vi "LuaVIEW Pull (refnum).vi"(5 "LuaVIEW reference in":T1, 11 "error in (no error)":errorcluster) -> (4 "refnum":refnum<vi>, 6 "LuaVIEW reference out":T1, 15 "error out":errorcluster)   [LabVIEW 2013]
doc: "Retrieves a refnum data item from the head/bottom of the Lua stack and removes it, thereby shifting any remaining data items down by one. The returned value is a generic refnum that identifies some LabVIEW side object and must be cast to the appropriate type before use. This VI is part of a polymorphic set that supports the pulling various data types. To change the type being pulled, pop up on this VI's diagram icon and use the \"Select Type\" sub menu."
uses:
  typedefs/t_LuaVIEW Reference.ctl
  typedefs/et_LuaVIEW CIN Actions.ctl
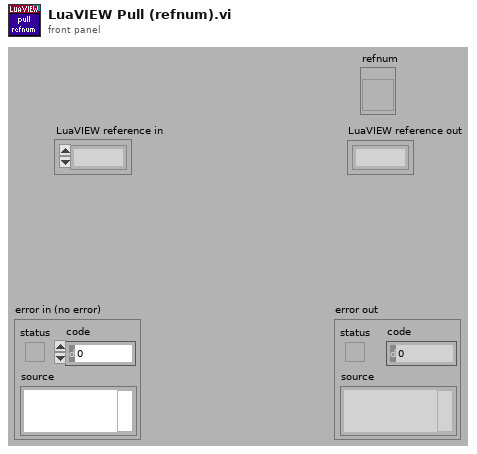
[diagram p1: front panel]
types:
  T1 = typedef "t_LuaVIEW Reference.ctl" = refnum<k1>
  T2 = typedef "et_LuaVIEW CIN Actions.ctl" = enum16{"checksynopsis", "_open", "_registerpublic", "_registerexport", "__never_an_error_result_ns", "luaversion", "cinversion", "_totals", "_taskcount", "pathological", "_unregnextpublic", "registryusecount", "__per_state_actions", "regsetprivate", "regsetindex", "regsetmodule", "_revokeexports", "_usepublic", "prepare", "compile", "execute", "call", "unregstaterefs", "_close", "pullboolean", "pullnumber", "pullI8", "pullU8", "pullI16", "pullU16", "pullI32", "pullU32", "pullobject", "pullrefnum", "pullstring", "pullflat", "pushflat", "pushobject", "getattribute", "setattribute", "stacktostring", "_startyieldtest", "_endyieldtest", "_pollprintbuffer", "__never_an_error_result_ps", "_pollexport", "setclone", "forcecleanup", "gettop", "clearstack", "insert", "pushboolean", "pushnumber", "pushrefnum", "pushstring", "pushnil", "pushvalue", "gettaskref", "settaskref"}
  T3 = typedef "et_LuaVIEW CIN Results.ctl" = enum16{"OK", "error", "main", "call", "clonecall", "modulecall", "exportcall", "index", "yield"}
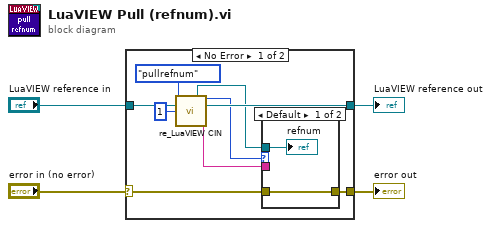
[diagram p0: block diagram]
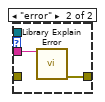
[diagram p2: hidden frame]
diagram:
  n1 = case shown="No Error" "error in (no error)" {
    selector: "error in (no error)" -> [w8 w19]
    tunnel: [w10 w18] -> w2
    tunnel: [w9 w19] -> w1
    tunnel: "LuaVIEW reference in" -> [w12 w18]
    frame No Error {
      n2 = call "re_LuaVIEW CIN.vi"("action"=et_LuaVIEW_CIN_Actions."pullrefnum", "LuaVIEW reference in"=w12, "index in"=1) -> ("refnum out"=w5:refnum<vi>, "result"=w7:T3, "LuaVIEW reference out"=w10:T1, "string out"=w6:string)  [unwired: 6 in, 3 out]
      n3 = case shown="Default" w7 {
        tunnel: w6 -> [_ w17]
        tunnel: [w15 w16] -> w9
        tunnel: w8 -> [w15 _]
        tunnel: w5 -> [w14 _]
        frame Default {
          "refnum" <- w14
        }
        frame "error" {
          n4 = call "Library Explain Error.vi"("explanation prefix (none)"=w17) -> ("explained error"=w16:errorcluster)  [unwired: 14 in]
        }
      }
    }
    frame Error {
    }
  }
  "LuaVIEW reference out" <- w2
  "error out" <- w1
